vi "Navigation_Main_derping_stuff_up 5thv2.vi"() -> ()   [LabVIEW 2015]
uses:
  <vilib>/myRIO/Common/Instrument Driver Framework/Utilities/typedefs/Generic FPGA Reference.ctl
  <vilib>/myRIO/Common/Instrument Driver Framework/Utilities/typedefs/myRIO v1.0 Reference.ctl
  <vilib>/myRIO/Common/Instrument Driver Framework/Utilities/typedefs/Hardware Version Enum.ctl
  <vilib>/myRIO/Common/Instrument Driver Framework/Utilities/typedefs/myRIO Generic Hardware Reference.ctl
  <vilib>/userdefined/High Color/nirio_resource_hc.ctl
  <vilib>/myRIO/Instrument Drivers/Onboard IO/PWM/typedefs/PWM Configuration.ctl
  <vilib>/myRIO/Instrument Drivers/Onboard IO/PWM/PWM.lvlib
  <vilib>/myRIO/Common/Instrument Driver Framework/myRIO v1.0/PWM/typedefs/PWM Channels Enum.ctl
  <vilib>/myRIO/Instrument Drivers/Onboard IO/PWM/typedefs/PWM Reference.ctl
  <vilib>/myRIO/Instrument Drivers/Onboard IO/PWM/vis/myRIO PWM Open.xnode
  <vilib>/myRIO/Common/Instrument Driver Framework/myRIO v1.0/PWM/vis/myRIO v1.1 Open PWM.vi
  <vilib>/rvi/interface/nirviOpenFPGA/nirviOpenFPGA.xnode
  <vilib>/myRIO/Instrument Drivers/Utilities/Utilities.lvlib
  <vilib>/rvi/interface/nirviReadWriteControl/nirviReadWriteControl.xnode
  <vilib>/rvi/interface/Simulation/niFpgaSimulationCallBeginRW.vi
  <vilib>/rvi/errors/niLvFpgaAdjustHostInterfaceError.vi
  UNCC_AST2_Master/FPGA Bitfiles/NavigationProjec_FPGATarget2_FPGAMainNavigati_PWPHW8gwDxI.lvbitx
  <vilib>/addons/control/pid/NI_PID_pid.lvlib
  <vilib>/addons/control/pid/pid.llb/PID (DBL).vi
  <vilib>/FPGAPlugInAG/myRIO-1900/niLvFpga_Open_myRIO-1900.vi
  <vilib>/rvi/interface/common/dynamic/niFpgaDynamicAddResources.vi
panel:
  out "x/y":dbl
  out "scale":dbl=1.0
  in  "x goal":dbl=20.0
  out "left":dbl
  out "right":dbl
  out "actual pwm left":dbl
  in  "stop 3":bool
  out "left pwm":dbl(graph)
  out "dt out (s) left":dbl format="%.3f"
  in  "output range 3":cluster{"output high":dbl, "output low":dbl}={"output high"=0.13333, "output low"=-0.13333} {"output low" format="%.6f"; "output high" format="%.5f"}
  in  "PID gains 3":T1={"proportional gain (Kc)"=0.002, "integral time (Ti, min)"=7e-07, "derivative time (Td, min)"=0.0} {"derivative time (Td, min)" format="%.8f"; "integral time (Ti, min)" format="%.8f"; "proportional gain (Kc)" format="%.8f"}
  out "desired pwm 2":dbl
  out "feedback 2":dbl
  out ".not. x? 3":bool
  out "Elapsed Time (s) 2":dbl caption="Elapsed Time (s)"
  out "x traveled 2":dbl
  out "y traveled 2":dbl
  out "avg left":dbl
  out "avg right":dbl
  out "psi dot 2":dbl
  out "distance traveled 2":dbl
  out "y dot 2":dbl
  out "x dot 2":dbl
  out "x position 2":dbl
  out "y position 2":dbl
  out "reset x y 2":dbl
  out "Tick Count(mSec) 2":u32 caption="Tick Count(mSec)"
  in  "start y 2":dbl=3.0
  in  "start x 2":dbl=1.0
  in  "start y":dbl=3.0
  in  "start x":dbl=1.0
  out "actual pwm right":dbl
  in  "stop 2":bool
  out "right pwm":dbl(graph)
  out "dt out (s) right":dbl format="%.3f"
  in  "output range 2":cluster{"output high":dbl, "output low":dbl}={"output high"=0.13333, "output low"=-0.13333} {"output low" format="%.6f"; "output high" format="%.5f"}
  in  "PID gains 2":T1={"proportional gain (Kc)"=0.002, "integral time (Ti, min)"=7e-07, "derivative time (Td, min)"=0.0} {"derivative time (Td, min)" format="%.8f"; "integral time (Ti, min)" format="%.8f"; "proportional gain (Kc)" format="%.8f"}
  out "desired pwm":dbl
  out "feedback right":dbl
  out ".not. x? 2":bool
  out "Elapsed Time (s)":dbl
  out "LF Rot Velocity (rot/s)":dbl
  out "LM Rot Velocity (rot/s)":dbl
  out "LR Rot Velocity (rot/s)":dbl
  out "RR Rot Velocity (rot/s)":dbl
  out "RM Linear Velocity (rot/s)":dbl
  out "RF Linear Velocity (rot/s)":dbl
  in  "Encoder Reset":bool
  out "SYS.SELECTA":u8 format="%08b"
  out "ENC.B_c.CNTR":i32
  out "ENC.B_b.CNTR":i32
  out "ENC.B_a.CNTR":i32
  out "ENC.A_c.CNTR":i32
  out "ENC.A_b.CNTR":i32
  out "ENC.A_a.CNTR":i32
  in  "R Min Linear Velocity (ft/s)":dbl=-2.0 format="%#_13g"
  in  "R Max Linear Velocity (ft/s)":dbl=2.0 format="%#_13g"
  in  "L Min Linear Velocity (ft/s)":dbl=-2.0 format="%#_13g"
  in  "L Max Linear Velocity (ft/s)":dbl=2.0 format="%#_13g"
  out "Current Rot Velocity (rot/s)":T2(graph)
  # "Motor Control Parameters"
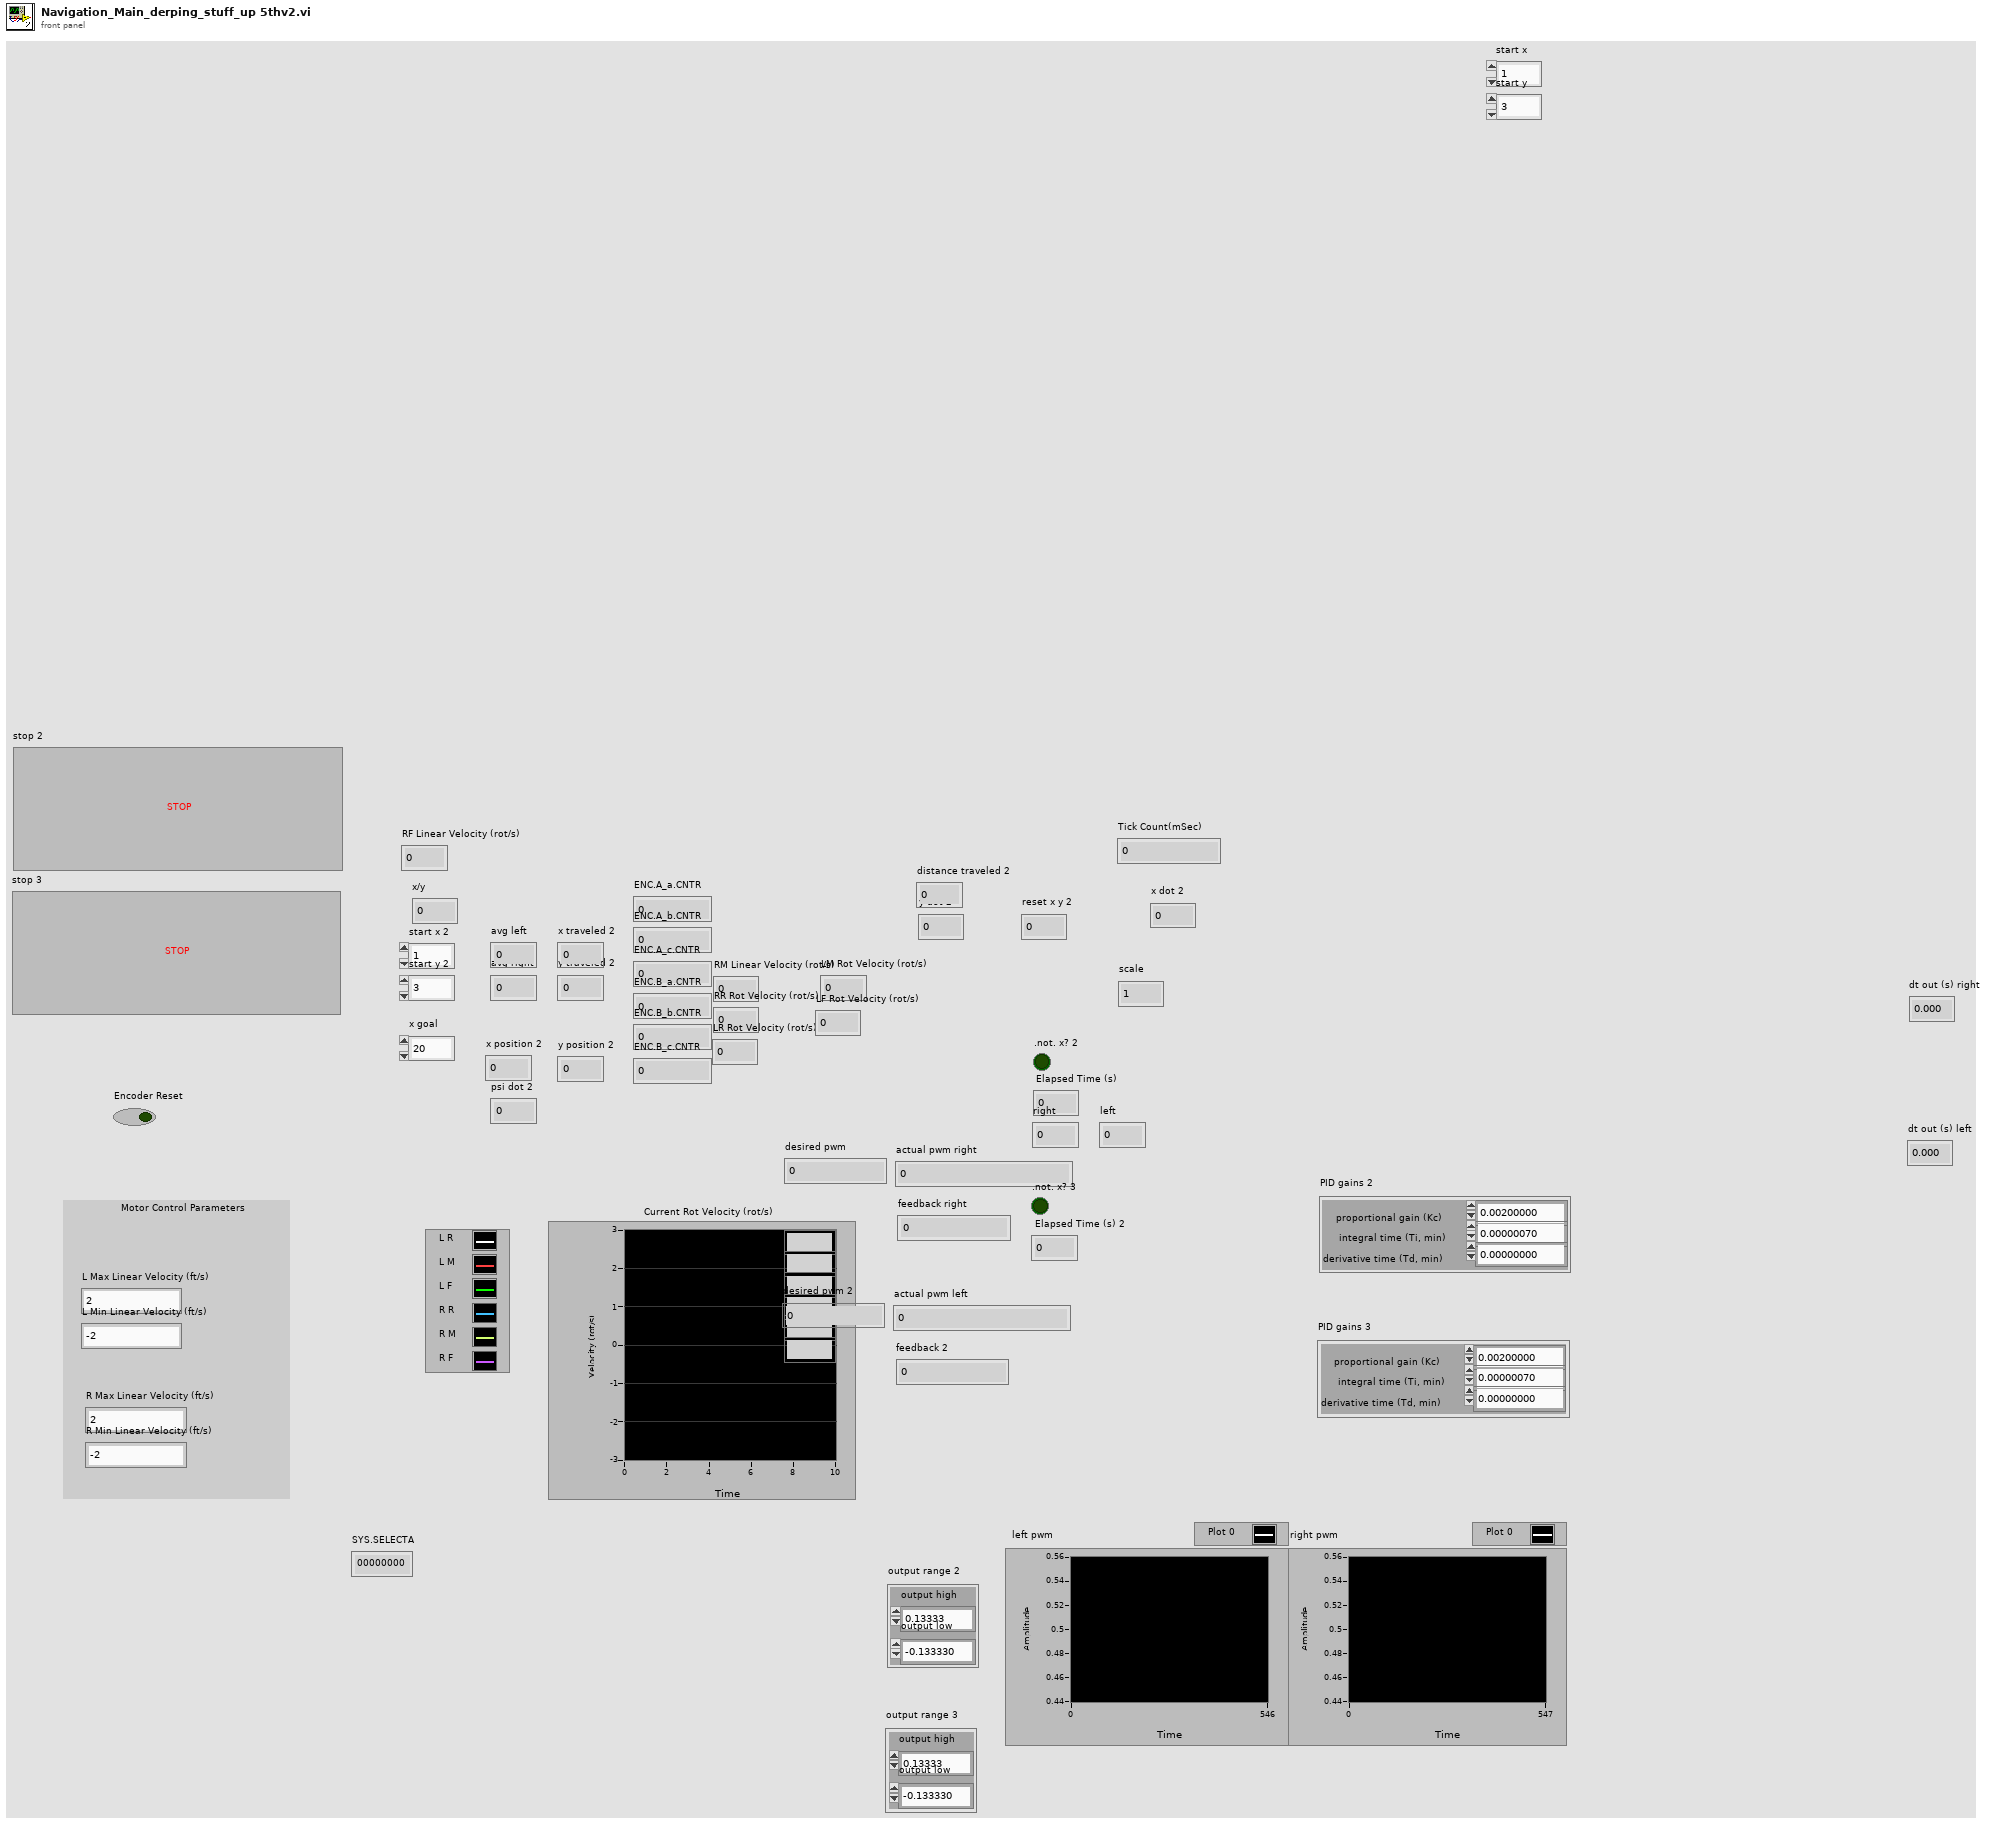
[diagram p1: front panel]
types:
  T1 = cluster{"proportional gain (Kc)":dbl, "integral time (Ti, min)":dbl, "derivative time (Td, min)":dbl}
  T2 = cluster{"Rotational Velocity (RPS)":dbl, "Rotational Velocity (RPS)":dbl, "Rotational Velocity (RPS)":dbl, "Rotational Velocity (RPS)":dbl, "Rotational Velocity (RPS)":dbl, "Rotational Velocity (RPS)":dbl}
  T3 = typedef "nirio_resource_hc.ctl" = tag
  T4 = typedef "Hardware Version Enum.ctl" = enum16{"Unknown", "myRIO-1900", "myRIO-1950", "roboRIO"}
  T5 = typedef "PWM.lvlib/PWM Reference.ctl" = cluster{"myRIO Reference":T6, "PWM Channels Enum":T9, "PWM Configuration":T10}
  T6 = typedef "myRIO Generic Hardware Reference.ctl" = cluster{"myRIO Model":T4, "myRIO Hardware Reference":T7}
  T7 = typedef "myRIO v1.0 Reference.ctl" = cluster{"Generic FPGA Reference":T8, "Allow multiple opens":bool}
  T8 = typedef "Generic FPGA Reference.ctl" = refnum<k20>
  T9 = typedef "PWM Channels Enum.ctl" = enum16{"Not Connected", "C/PWM0", "C/PWM1", "A/PWM0", "A/PWM1", "A/PWM2", "B/PWM0", "B/PWM1", "B/PWM2", "PWM/PWM0", "PWM/PWM1", "PWM/PWM2", "PWM/PWM3", "PWM/PWM4", "PWM/PWM5", "PWM/PWM6", "PWM/PWM7", "PWM/PWM8", "PWM/PWM9"}
  T10 = typedef "PWM.lvlib/PWM Configuration.ctl" = cluster{"Frequency":dbl, "Duty Cycle":dbl}
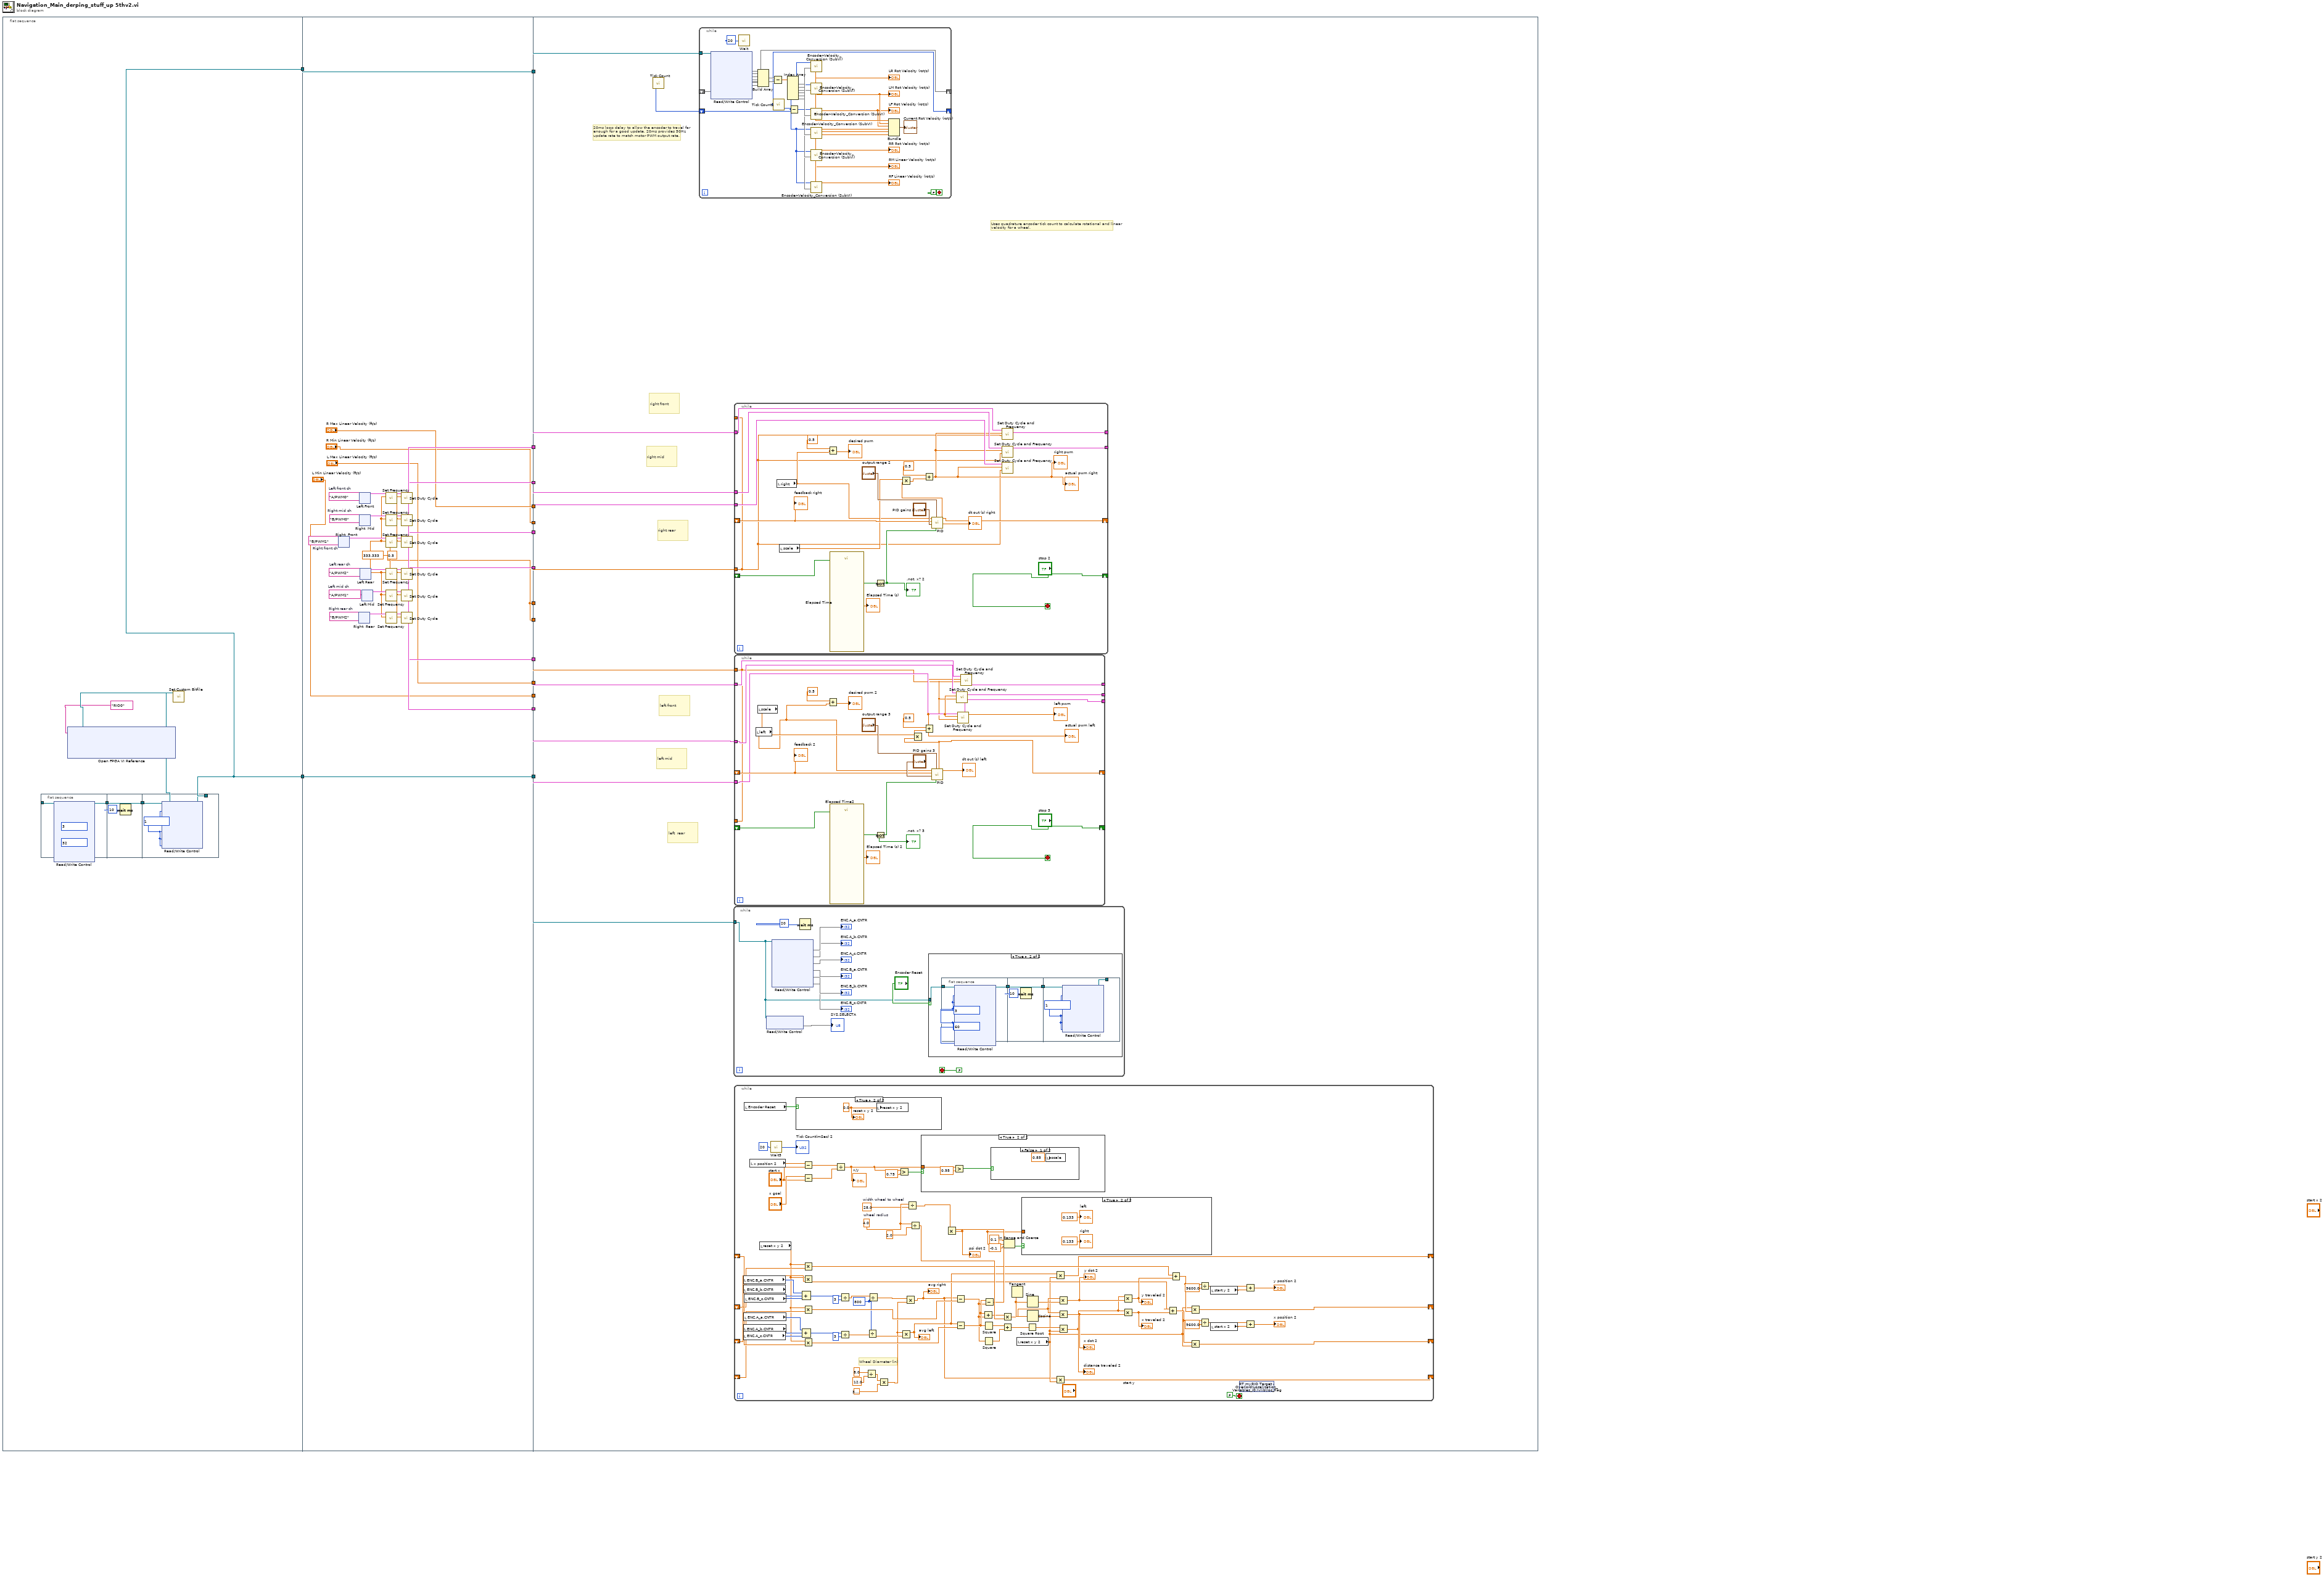
[diagram p0: block diagram]
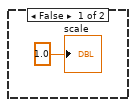
[diagram p2: hidden frame]
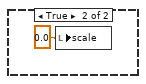
[diagram p3: hidden frame]
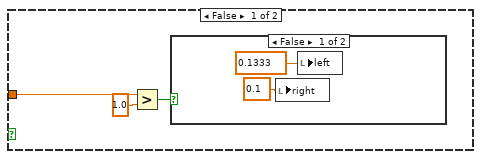
[diagram p4: hidden frame]
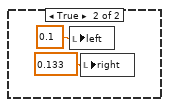
[diagram p5: hidden frame]
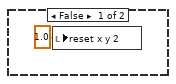
[diagram p6: hidden frame]
diagram:
  n1 = flat-sequence {
    tunnel: [w19] -> w4
    tunnel: [w19] -> w2
    tunnel: [w32] -> w16
    tunnel: [w47] -> w15
    tunnel: [w43] -> w14
    tunnel: [w42] -> w13
    tunnel: [w41] -> w12
    tunnel: [w40] -> w11
    tunnel: [w39] -> w10
    tunnel: ["L Max Linear Velocity (ft/s)"] -> w9
    tunnel: ["L Min Linear Velocity (ft/s)"] -> w8
    tunnel: ["R Max Linear Velocity (ft/s)"] -> w7
    tunnel: ["R Min Linear Velocity (ft/s)"] -> w6
    tunnel: [w34] -> w5
    tunnel: w4 -> [w33]
    tunnel: [w33] -> w3
    tunnel: w2 -> [w34]
    tunnel: [w32] -> w1
    tunnel: w16 -> [_]
    tunnel: w15 -> [w160]
    tunnel: w14 -> [w166]
    tunnel: w13 -> [w162]
    tunnel: w12 -> [w163]
    tunnel: w11 -> [w161]
    tunnel: w10 -> [w165]
    tunnel: w9 -> [_]
    tunnel: w8 -> [_]
    tunnel: w7 -> [_]
    tunnel: w6 -> [_]
    tunnel: w5 -> [w168]
    tunnel: w3 -> [w167]
    tunnel: w1 -> [w164]
    frame #0 {
      n2 = flat-sequence {
        tunnel: w20 -> [w25]
        tunnel: [w23] -> w22
        tunnel: w22 -> [w27]
        tunnel: [w27] -> w21
        tunnel: w21 -> [w30]
        tunnel: [w29] -> w19
        frame #0 {
          w24 = u8 32 ("SYS.SELECTA")
          w26 = u8 3 ("ENC.B_c.CNFG")
          n3 = xnode "Read/Write Control"("FPGA VI Reference In"=w25, "ENC.A_a.CNFG"=w26, "ENC.A_b.CNFG"=w26, "ENC.A_c.CNFG"=w26, "ENC.B_a.CNFG"=w26, "ENC.B_b.CNFG"=w26, "ENC.B_c.CNFG"=w26, "SYS.SELECTA"=w24, "SYS.SELECTB"=w24) -> ("FPGA VI Reference Out"=w23:refnum<k20>)  [unwired: 1 in, 1 out]
        }
        frame #1 {
          n4 = Wait (ms)(milliseconds to wait=u32 10) -> ()  [unwired: 1 out]
        }
        frame #2 {
          w31 = u8 1 ("ENC.B_c.CNFG")
          n5 = xnode "Read/Write Control"("FPGA VI Reference In"=w30, "ENC.A_a.CNFG"=w31, "ENC.A_b.CNFG"=w31, "ENC.A_c.CNFG"=w31, "ENC.B_a.CNFG"=w31, "ENC.B_b.CNFG"=w31, "ENC.B_c.CNFG"=w31) -> ("FPGA VI Reference Out"=w29:refnum<k20>)  [unwired: 1 in, 1 out]
        }
      }
      n6 = xnode "Open FPGA VI Reference"("resource name"=tag "RIO0") -> ("FPGA VI Reference Out"=w18:refnum<k20>)  [unwired: 1 in, 1 out]
      n7 = call <vilib>:"Set Custom Bitfile.vi"("Custom FPGA Reference In"=w18) -> ("Custom FPGA Reference Out"=w20:refnum<k20>)  [unwired: 9 in, 1 out]
    }
    frame #1 {
      w44 = 0.5 ("Duty Cycle")
      w32 = 333.333 ("Frequency [Hz]")
      w58 = tag "B/PWM2"  # Right rear ch
      w59 = tag "B/PWM0"  # Right mid ch
      w60 = tag "B/PWM1"  # Right front ch
      w61 = tag "A/PWM2"  # Left rear ch
      w62 = tag "A/PWM1"  # Left mid ch
      w63 = tag "A/PWM0"  # Left front ch
      n8 = xnode "Right  Front"("Channel Name"=w60) -> ("PWM Ref Out"=w54:T5)  [unwired: 2 in, 1 out]
      n9 = xnode "Right  Rear"("Channel Name"=w58) -> ("PWM Ref Out"=w52:T5)  [unwired: 2 in, 1 out]
      n10 = xnode "Left Front"("Channel Name"=w63) -> ("PWM Ref Out"=w57:T5)  [unwired: 2 in, 1 out]
      n11 = xnode "Right  Mid"("Channel Name"=w59) -> ("PWM Ref Out"=w53:T5)  [unwired: 2 in, 1 out]
      n12 = xnode "Left Rear"("Channel Name"=w61) -> ("PWM Ref Out"=w55:T5)  [unwired: 2 in, 1 out]
      n13 = xnode "Left Mid"("Channel Name"=w62) -> ("PWM Ref Out"=w56:T5)  [unwired: 2 in, 1 out]
      n14 = call <vilib>:"Set Frequency.vi"("Frequency [Hz]"=w32, "PWM Ref In"=w57) -> ("PWM Ref Out"=w51:T5)  [unwired: 7 in, 1 out]
      n15 = call <vilib>:"Set Frequency.vi"("Frequency [Hz]"=w32, "PWM Ref In"=w53) -> ("PWM Ref Out"=w49:T5)  [unwired: 7 in, 1 out]
      n16 = call <vilib>:"Set Frequency.vi"("Frequency [Hz]"=w32, "PWM Ref In"=w54) -> ("PWM Ref Out"=w48:T5)  [unwired: 7 in, 1 out]
      n17 = call <vilib>:"Set Frequency.vi"("Frequency [Hz]"=w32, "PWM Ref In"=w55) -> ("PWM Ref Out"=w46:T5)  [unwired: 7 in, 1 out]
      n18 = call <vilib>:"Set Frequency.vi"("Frequency [Hz]"=w32, "PWM Ref In"=w56) -> ("PWM Ref Out"=w45:T5)  [unwired: 7 in, 1 out]
      n19 = call <vilib>:"Set Frequency.vi"("Frequency [Hz]"=w32, "PWM Ref In"=w52) -> ("PWM Ref Out"=w50:T5)  [unwired: 7 in, 1 out]
      n20 = call <vilib>:"Set Duty Cycle.vi"("Duty Cycle"=w44, "PWM Ref In"=w51) -> ("PWM Ref Out"=w39:T5)  [unwired: 7 in, 1 out]
      n21 = call <vilib>:"Set Duty Cycle.vi"("Duty Cycle"=w44, "PWM Ref In"=w49) -> ("PWM Ref Out"=w42:T5)  [unwired: 7 in, 1 out]
      n22 = call <vilib>:"Set Duty Cycle.vi"("Duty Cycle"=w44, "PWM Ref In"=w48) -> ("PWM Ref Out"=w43:T5)  [unwired: 7 in, 1 out]
      n23 = call <vilib>:"Set Duty Cycle.vi"("Duty Cycle"=w44, "PWM Ref In"=w46) -> ("PWM Ref Out"=w47:T5)  [unwired: 7 in, 1 out]
      n24 = call <vilib>:"Set Duty Cycle.vi"("Duty Cycle"=w44, "PWM Ref In"=w45) -> ("PWM Ref Out"=w40:T5)  [unwired: 7 in, 1 out]
      n25 = call <vilib>:"Set Duty Cycle.vi"("Duty Cycle"=w44, "PWM Ref In"=w50) -> ("PWM Ref Out"=w41:T5)  [unwired: 7 in, 1 out]
    }
    frame #2 {
      # "left  rear"
      # "left mid"
      # "left front"
      # "right rear"
      # "right mid"
      # "right front"
      # "Uses quadrature encoder tick count to calculate rotational and linear velocity for a wheel."
      # "20ms loop delay to allow the encoder to travel far enough for a good update. 20ms provides 50Hz update rate to match motor PWM output rate."
      n26 = call "Tick Count"() -> ("Tick Count(uSec)"=w169:u32)
      n27 = while {
        shift-right: [w359] -> _
        shift-left: _ -> [w358]
        shift-right: [w356] -> _
        shift-left: w169 -> [w355]
        tunnel: w167 -> [w366]
        stop <- FALSE stop-if-true
        n28 = xnode "Read/Write Control"("FPGA VI Reference In"=w366) -> ("ENC.A_a.CNTR"=w365, "ENC.A_b.CNTR"=w364, "ENC.A_c.CNTR"=w363, "ENC.B_a.CNTR"=w362, "ENC.B_b.CNTR"=w361, "ENC.B_c.CNTR"=w360)  [unwired: 1 in, 2 out]
        n29 = call "Wait"("Count(mSec)"=u32 20) -> ()  [unwired: 1 out]
        n30 = Build Array(w365, w364, w363, w362, w361, w360) -> (w359:void[])
        n31 = Subtract(x=w359, y=w358) -> (x-y=w357:dbl)
        n32 = call "Tick Count2"() -> ("Tick Count(uSec)"=w356:u32)
        n33 = Index Array(array=w357) -> (element #1=w354, element #2=w353, element #3=w352, element #4=w351, element #5=w350, element #6=w349)  [unwired: 6 in]
        n34 = Subtract(x=w356, y=w355) -> (x-y=w348:u32)
        n35 = call "Encoder-Velocity_Conversion (SubVI).vi"("delta  Encoder Count"=w353, "dt (uSec)"=w348) -> ("Rotational Velocity (RPS)"=w343:dbl)  [unwired: 7 in, 2 out]
        "LM Rot Velocity (rot/s)" <- w343
        n36 = call "Encoder-Velocity_Conversion (SubVI).vi"("delta  Encoder Count"=w352, "dt (uSec)"=w348) -> ("Rotational Velocity (RPS)"=w342:dbl)  [unwired: 7 in, 2 out]
        "LF Rot Velocity (rot/s)" <- w342
        n37 = call "Encoder-Velocity_Conversion (SubVI).vi"("delta  Encoder Count"=w354, "dt (uSec)"=w348) -> ("Rotational Velocity (RPS)"=w344:dbl)  [unwired: 7 in, 2 out]
        "LR Rot Velocity (rot/s)" <- w344
        n38 = call "Encoder-Velocity_Conversion (SubVI).vi"("delta  Encoder Count"=w351, "dt (uSec)"=w348) -> ("Rotational Velocity (RPS)"=w341:dbl)  [unwired: 7 in, 2 out]
        "RR Rot Velocity (rot/s)" <- w341
        n39 = call "Encoder-Velocity_Conversion (SubVI).vi"("delta  Encoder Count"=w350, "dt (uSec)"=w348) -> ("Rotational Velocity (RPS)"=w345:dbl)  [unwired: 7 in, 2 out]
        "RM Linear Velocity (rot/s)" <- w345
        n40 = call "Encoder-Velocity_Conversion (SubVI).vi"("delta  Encoder Count"=w349, "dt (uSec)"=w348) -> ("Rotational Velocity (RPS)"=w346:dbl)  [unwired: 7 in, 2 out]
        "RF Linear Velocity (rot/s)" <- w346
        n41 = Bundle("Rotational Velocity (RPS)"=w344, "Rotational Velocity (RPS)"=w343, "Rotational Velocity (RPS)"=w342, "Rotational Velocity (RPS)"=w341, "Rotational Velocity (RPS)"=w345, "Rotational Velocity (RPS)"=w346) -> (→"Current Rot Velocity (rot/s)":T2)  [unwired: 1 in]
      }
      n42 = while {
        tunnel: w168 -> [w318]
        stop <- FALSE stop-if-true
        n43 = xnode "Read/Write Control"("FPGA VI Reference In"=w318) -> ("SYS.SELECTA"=→"SYS.SELECTA")  [unwired: 1 in, 2 out]
        n44 = xnode "Read/Write Control"("FPGA VI Reference In"=w318) -> ("ENC.A_a.CNTR"=→"ENC.A_a.CNTR", "ENC.A_b.CNTR"=→"ENC.A_b.CNTR", "ENC.A_c.CNTR"=→"ENC.A_c.CNTR", "ENC.B_a.CNTR"=→"ENC.B_a.CNTR", "ENC.B_b.CNTR"=→"ENC.B_b.CNTR", "ENC.B_c.CNTR"=→"ENC.B_c.CNTR")  [unwired: 1 in, 2 out]
        n45 = Wait (ms)(milliseconds to wait=u32 20) -> ()  [unwired: 1 out]
        n46 = case shown="True" "Encoder Reset" {
          tunnel: w318 -> [_ w329]
          frame False {
          }
          frame True {
            n47 = flat-sequence {
              tunnel: w329 -> [w334]
              tunnel: [w332] -> w331
              tunnel: w331 -> [w336]
              tunnel: [w336] -> w330
              tunnel: w330 -> [w339]
              tunnel: [w338] -> _
              frame #0 {
                w333 = u8 60 ("SYS.SELECTA")
                w335 = u8 3 ("ENC.B_c.CNFG")
                n48 = xnode "Read/Write Control"("FPGA VI Reference In"=w334, "ENC.A_a.CNFG"=w335, "ENC.A_b.CNFG"=w335, "ENC.A_c.CNFG"=w335, "ENC.B_a.CNFG"=w335, "ENC.B_b.CNFG"=w335, "ENC.B_c.CNFG"=w335, "SYS.SELECTA"=w333, "SYS.SELECTB"=w333) -> ("FPGA VI Reference Out"=w332:refnum<k20>)  [unwired: 1 in, 1 out]
              }
              frame #1 {
                n49 = Wait (ms)(milliseconds to wait=u32 10) -> ()  [unwired: 1 out]
              }
              frame #2 {
                w340 = u8 1 ("ENC.B_c.CNFG")
                n50 = xnode "Read/Write Control"("FPGA VI Reference In"=w339, "ENC.A_a.CNFG"=w340, "ENC.A_b.CNFG"=w340, "ENC.A_c.CNFG"=w340, "ENC.B_a.CNFG"=w340, "ENC.B_b.CNFG"=w340, "ENC.B_c.CNFG"=w340) -> ("FPGA VI Reference Out"=w338:refnum<k20>)  [unwired: 1 in, 1 out]
              }
            }
          }
        }
      }
      n51 = while {
        tunnel: w166 -> [w316]
        tunnel: [w317] -> _
        tunnel: [w295] -> _
        shift-right: [w302] -> _
        shift-left: _ -> [w312]
        shift-right: ["stop 2"] -> _
        shift-left: _ -> [w307]
        tunnel: w164 -> [w295]
        tunnel: w163 -> [w297]
        tunnel: w162 -> [w299]
        tunnel: [w298] -> _
        stop <- "stop 2" stop-if-true
        n52 = local read "right"() -> (w300:dbl)
        n53 = local read "scale"() -> (w303:dbl)
        n54 = Add(x=0.5, y=w300) -> (x+y=→"desired pwm":dbl)
        n55 = call "Elapsed Time"("Reset"=w307) -> ("Elapsed Time (s)"=→"Elapsed Time (s)":dbl, "Time has Elapsed"=w310:bool)  [unwired: 11 in, 6 out]
        n56 = Not(x=w310) -> (.not. x?=w309:bool)
        ".not. x? 2" <- w309
        n57 = call-poly <vilib>:"PID.vi"("reinitialize? (F)"=w309, "output range"="output range 2", "PID gains"="PID gains 2", "process variable"=w312, "setpoint"=w300) -> ("dt out (s)"=→"dt out (s) right":dbl, "output"=w302:dbl)  [unwired: 5 in]
        n58 = Multiply(x=w303, y=w302) -> (x*y=w301:dbl)
        n59 = Add(x=0.5, y=w301) -> (x+y=w296:dbl)
        "actual pwm right" <- w296
        "right pwm" <- w296
        n60 = call <vilib>:"Set Duty Cycle and Frequency.vi"("Frequency [Hz]"=w295, "Duty Cycle"=w296, "PWM Ref In"=w316) -> ("PWM Ref Out"=w317:T5)  [unwired: 6 in, 1 out]
        n61 = call <vilib>:"Set Duty Cycle and Frequency.vi"("Frequency [Hz]"=w295, "Duty Cycle"=w296, "PWM Ref In"=w299) -> ("PWM Ref Out"=w298:T5)  [unwired: 6 in, 1 out]
        n62 = call <vilib>:"Set Duty Cycle and Frequency.vi"("Frequency [Hz]"=w295, "Duty Cycle"=w296, "PWM Ref In"=w297) -> ()  [unwired: 6 in, 2 out]
        "feedback right" <- w312
      }
      n63 = while {
        tunnel: w165 -> [w192]
        tunnel: [w193] -> _
        tunnel: w164 -> [w172]
        shift-right: [w178] -> _
        shift-left: _ -> [w188]
        shift-right: ["stop 3"] -> _
        shift-left: _ -> [w183]
        tunnel: [w172] -> _
        tunnel: w161 -> [w175]
        tunnel: w160 -> [w174]
        tunnel: [w171] -> _
        tunnel: [w170] -> _
        stop <- "stop 3" stop-if-true
        n64 = local read "left"() -> (w176:dbl)
        n65 = local read "scale"() -> (w179:dbl)
        n66 = Add(x=0.5, y=w176) -> (x+y=→"desired pwm 2":dbl)
        n67 = call "Elapsed Time2"("Reset"=w183) -> ("Elapsed Time (s)"=→"Elapsed Time (s) 2":dbl, "Time has Elapsed"=w186:bool)  [unwired: 11 in, 6 out]
        n68 = Not(x=w186) -> (.not. x?=w185:bool)
        ".not. x? 3" <- w185
        n69 = call-poly <vilib>:"PID.vi"("reinitialize? (F)"=w185, "output range"="output range 3", "PID gains"="PID gains 3", "process variable"=w188, "setpoint"=w176) -> ("dt out (s)"=→"dt out (s) left":dbl, "output"=w178:dbl)  [unwired: 5 in]
        n70 = Multiply(x=w179, y=w178) -> (x*y=w177:dbl)
        n71 = Add(x=0.5, y=w177) -> (x+y=w173:dbl)
        "actual pwm left" <- w173
        "left pwm" <- w173
        n72 = call <vilib>:"Set Duty Cycle and Frequency.vi"("Frequency [Hz]"=w172, "Duty Cycle"=w173, "PWM Ref In"=w175) -> ("PWM Ref Out"=w171:T5)  [unwired: 6 in, 1 out]
        n73 = call <vilib>:"Set Duty Cycle and Frequency.vi"("Frequency [Hz]"=w172, "Duty Cycle"=w173, "PWM Ref In"=w174) -> ("PWM Ref Out"=w170:T5)  [unwired: 6 in, 1 out]
        n74 = call <vilib>:"Set Duty Cycle and Frequency.vi"("Frequency [Hz]"=w172, "Duty Cycle"=w173, "PWM Ref In"=w192) -> ("PWM Ref Out"=w193:T5)  [unwired: 6 in, 1 out]
        "feedback 2" <- w188
      }
      n75 = while {
        shift-right: [w228] -> _
        shift-left: _ -> [w265]
        shift-right: [w225] -> _
        shift-left: _ -> [w264]
        shift-right: [w227] -> _
        shift-left: _ -> [w240]
        shift-right: [w226] -> _
        shift-left: _ -> [w239]
        stop <- FALSE stop-if-true
        w197 = 800 ("y")
        w261 = 28.0  # width wheel to wheel
        w262 = 4.0  # wheel radius
        # "Wheel Diameter (in)"
        n76 = local read "ENC.B_a.CNTR"() -> (w269:i32)
        n77 = local read "ENC.B_b.CNTR"() -> (w268:i32)
        n78 = local read "ENC.A_b.CNTR"() -> (w271:i32)
        n79 = local read "ENC.A_c.CNTR"() -> (w270:i32)
        n80 = local read "ENC.A_a.CNTR"() -> (w272:i32)
        n81 = local read "Encoder Reset"() -> (w221:bool)
        n82 = local read "ENC.B_c.CNTR"() -> (w267:i32)
        n83 = local read "x position 2"() -> (w213:dbl)
        n84 = local read "reset x y 2"() -> (w224:dbl)
        n85 = call "Wait3"("Count(mSec)"=u32 20) -> ("Tick Count(mSec)"=→"Tick Count(mSec) 2":u32)
        n86 = case shown="True" w221 {
          frame False {
            n87 = local write "reset x y 2"(1.0) -> ()
          }
          frame True {
            w294 = 0.0
            n88 = local write "reset x y 2"(w294) -> ()
            "reset x y 2" <- w294
          }
        }
        n89 = Compound Arithmetic op=ADD(w269, w268, w267) -> (w275:i32)
        n90 = Compound Arithmetic op=ADD(w272, w271, w270) -> (w276:i32)
        n91 = Subtract(x=w213, y="start x") -> (x-y=w207:dbl)
        n92 = Subtract(x="x goal", y="start x") -> (x-y=w206:dbl)
        n93 = Multiply(x=w224, y=w240) -> (x*y=w231:dbl)
        n94 = Multiply(x=w224, y=w239) -> (x*y=w230:dbl)
        n95 = Multiply(x=w224, y=w264) -> (x*y=w229:dbl)
        n96 = Multiply(x=w224, y=w265) -> (x*y=w232:dbl)
        n97 = Divide(x=w207, y=w206) -> (x/y=w210:dbl)
        "x/y" <- w210
        n98 = Divide(x=w275, y=3) -> (x/y=w200:dbl)
        n99 = Divide(x=w276, y=3) -> (x/y=w198:dbl)
        n100 = Divide(x=8.0, y=12.0) -> (x/y=w202:dbl)
        n101 = Divide(x=w197, y=w198) -> (x/y=w199:dbl)
        n102 = Divide(x=w200, y=w197) -> (x/y=w201:dbl)
        n103 = Multiply(x=w202, y=3.141592653589793) -> (x*y=w195:dbl)
        n104 = Greater?(x=w210, y=0.75) -> (0:w211:bool)
        n105 = Multiply(x=w195, y=w199) -> (x*y=w196:dbl)
        "avg left" <- w196
        n106 = Multiply(x=w201, y=w195) -> (x*y=w194:dbl)
        "avg right" <- w194
        n107 = Divide(x=w262, y=w261) -> (x/y=w257:dbl)
        n108 = Divide(x=w262, y=2.0) -> (x/y=w260:dbl)
        n109 = case shown="True" w211 {
          tunnel: w210 -> [_ w281]
          frame False {
            "scale" <- 1.0
          }
          frame True {
            n110 = Greater?(x=w281, y=0.95) -> (0:w279:bool)
            n111 = case shown="False" w279 {
              frame False {
                n112 = local write "scale"(0.85) -> ()
              }
              frame True {
                n113 = local write "scale"(0.0) -> ()
              }
            }
          }
        }
        n114 = Subtract(x=w194, y=w229) -> (x-y=w254:dbl)
        n115 = Subtract(x=w196, y=w232) -> (x-y=w255:dbl)
        n116 = Add(x=w255, y=w254) -> (x+y=w259:dbl)
        n117 = Square(x=w255) -> (x^2=w252:dbl)
        n118 = Square(x=w254) -> (x^2=w253:dbl)
        n119 = Subtract(x=w255, y=w254) -> (x-y=w258:dbl)
        n120 = Multiply(x=w258, y=w257) -> (x*y=w214:dbl)
        "psi dot 2" <- w214
        n121 = Multiply(x=w259, y=w260) -> (x*y=w248:dbl)
        n122 = Add(x=w252, y=w253) -> (x+y=w251:dbl)
        n123 = In Range and Coerce(upper limit=0.1, x=w214, lower limit=-0.1) -> (In Range?=w215:bool)  [unwired: 1 out]
        n124 = Tangent() -> (0:w256:dbl)  [unwired: 1 in]
        n125 = local read "reset x y 2"() -> (w222:dbl)
        n126 = case shown="True" w215 {
          tunnel: w214 -> [w286 _]
          frame False {
            n127 = Greater?(x=w286, y=1.0) -> (0:w284:bool)
            n128 = case shown="False" w284 {
              frame False {
                n129 = local write "right"(0.1) -> ()
                n130 = local write "left"(0.1333) -> ()
              }
              frame True {
                n131 = local write "left"(0.1) -> ()
                n132 = local write "right"(0.133) -> ()
              }
            }
          }
          frame True {
            "right" <- 0.133
            "left" <- 0.133
          }
        }
        n133 = Square Root(x=w251) -> (sqrt(x)=w245:dbl)
        n134 = Sine(x=w256) -> (sin(x)=w250:dbl)
        n135 = Cosine(x=w256) -> (cos(x)=w249:dbl)
        n136 = Multiply(x=w196, y=w222) -> (x*y=w228:dbl)
        n137 = Multiply(x=w194, y=w222) -> (x*y=w225:dbl)
        n138 = Multiply(x=w248, y=w250) -> (x*y=w247:dbl)
        "y dot 2" <- w247
        n139 = Multiply(x=w248, y=w249) -> (x*y=w246:dbl)
        "x dot 2" <- w246
        n140 = Multiply(x=w245, y=w222) -> (x*y=w223:dbl)
        "distance traveled 2" <- w223
        n141 = Multiply(x=w223, y=w247) -> (x*y=w243:dbl)
        "y traveled 2" <- w243
        n142 = Multiply(x=w223, y=w246) -> (x*y=w244:dbl)
        "x traveled 2" <- w244
        n143 = Add(x=w230, y=w244) -> (x+y=w242:dbl)
        n144 = Add(x=w231, y=w243) -> (x+y=w234:dbl)
        n145 = Multiply(x=w222, y=w234) -> (x*y=w227:dbl)
        n146 = Multiply(x=w242, y=w222) -> (x*y=w226:dbl)
        n147 = Divide(x=w234, y=9600.0) -> (x/y=w238:dbl)
        n148 = Divide(x=w242, y=9600.0) -> (x/y=w237:dbl)
        n149 = local read "start y 2"() -> (w236:dbl)
        n150 = local read "start x 2"() -> (w235:dbl)
        n151 = shared-variable "RT myRIO Target - Overlord\\Localization_Variables_r0.lvlib\\loc_flag"() -> ()  [unwired: 1 in, 2 out]
        n152 = Add(x=w238, y=w236) -> (x+y=→"y position 2":dbl)
        n153 = Add(x=w237, y=w235) -> (x+y=→"x position 2":dbl)
      }
    }
  }
